vi "LVClass_CorrectionDataManager GetDiagnosticsSingularVector.vi"(0 "CorrectionDataManager in":refnum<class "CorrectionDataManager.lvclass">, 11 "error in (no error)":errorcluster) -> (4 "CorrectionDataManager out":refnum<class "CorrectionDataManager.lvclass">, 6 "ArrayOfSingularValues":dbl[](array[numeric]), 15 "error out":errorcluster)   [LabVIEW 2020, in "CorrectionDataManager.lvclass"]
doc: "Get vector of singular values.\n\n--------------------------------------------------------------------------------\n\n<B>corrdata_managerIn </B> : CorrDataManager object.\n<B>corrdata_managerOut </B> : CorrDataManager object.\n<B>singular_vector </B> : Array of influences, sorted in descending order.\n<B>ErrorIn </B> : Error\n<B>ErrorOut </B> : Error\n\n--------------------------------------------------------------------------------"
uses:
  CorrectionDataManager.lvclass
  CorrectionDataManager.lvclass/CorrectionDataManager.ctl
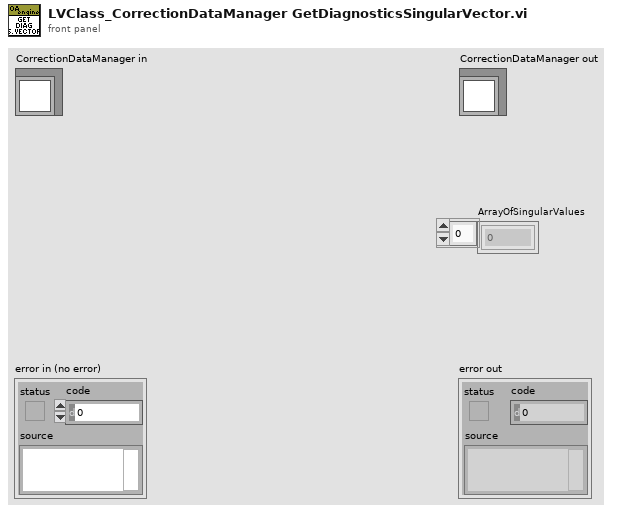
[diagram p1: front panel]
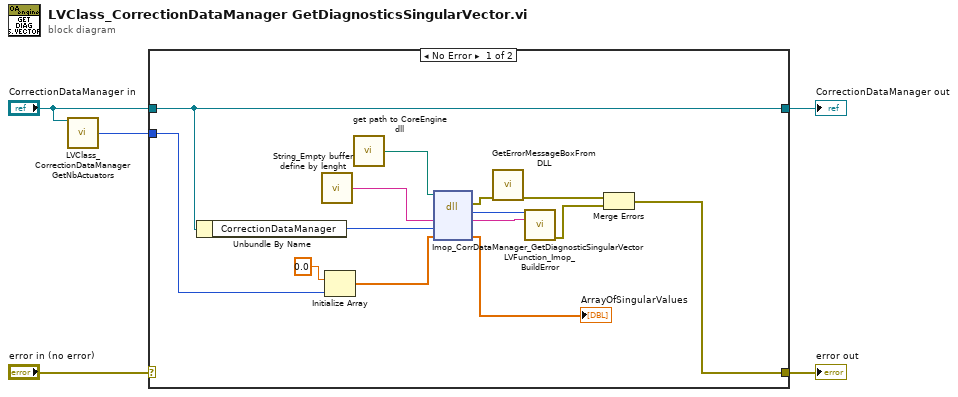
[diagram p0: block diagram]
diagram:
  n1 = call "LVClass_CorrectionDataManager GetNbActuators.vi"("CorrectionDataManager in"="CorrectionDataManager in") -> ("Nb actuators"=w1:i32)  [unwired: 12 in, 2 out]
  n2 = case shown="No Error" "error in (no error)" {
    selector: "error in (no error)" -> [_ w21]
    tunnel: [w11 w21] -> w4
    tunnel: [w12 w20] -> w5
    tunnel: "CorrectionDataManager in" -> [w12 w20]
    tunnel: w1 -> [w7 _]
    frame No Error {
      n3 = Unbundle By Name(w12) -> ("CorrectionDataManager"=w10:i32)
      n4 = call "String_Empty buffer define by lenght.vi"() -> ("Empty buffer"=w17:string)  [unwired: 1 in]
      n5 = Initialize Array(sgl 0.0, w7) -> (w6:sgl[])
      n6 = call "get path to CoreEngine dll.vi"() -> ("path to c_interface_vc100.dll"=w16:path)  [unwired: 12 in, 3 out]
      n7 = dll-call lib="D:/SOFTware/HASO_v3/SVN_trunk/ImOpCoreEngine4_LV2011/DLLs/c_interface_vc100.dll" fn="Imop_CorrDataManager_GetDiagnosticSingularVector"(path in=w16, "message"=w17, "WavefrontCorrection"=w10, "Singular_Vector"=w6) -> (error out=w15:errorcluster, "return type"=w19:i32, "message"=w18:string, "Singular_Vector"=→"ArrayOfSingularValues":sgl[])  [unwired: 3 in, 1 out]
      n8 = call "GetErrorMessageBoxFromDLL.vi"("error IN"=w15) -> ("error OUT"=w14:errorcluster)  [unwired: 10 in]
      n9 = call "LVFunction_Imop_BuildError.vi"("code"=w19, "String to Prepend to source (\"\")"=w18) -> ("error out"=w13:errorcluster)  [unwired: 13 in]
      n10 = Merge Errors(w14, w13) -> (w11:errorcluster)
    }
    frame Error {
    }
  }
  "error out" <- w4
  "CorrectionDataManager out" <- w5
